vi "BallShear_DependencyCheck.vi"(10 "Power":bool) -> (2 "Ready":bool)   [LabVIEW 2013]
uses:
  <vilib>/LabVIEW Interface for Arduino/LabVIEW Interface for Arduino.lvlib
panel:
  out "standard error":string
  out "standard output":string
  in  "Path to Script":path
  out "Command":string
  out "source":string
  out "code":i32
  out "status":bool
  in  "Errors":bool[](array[boolean])
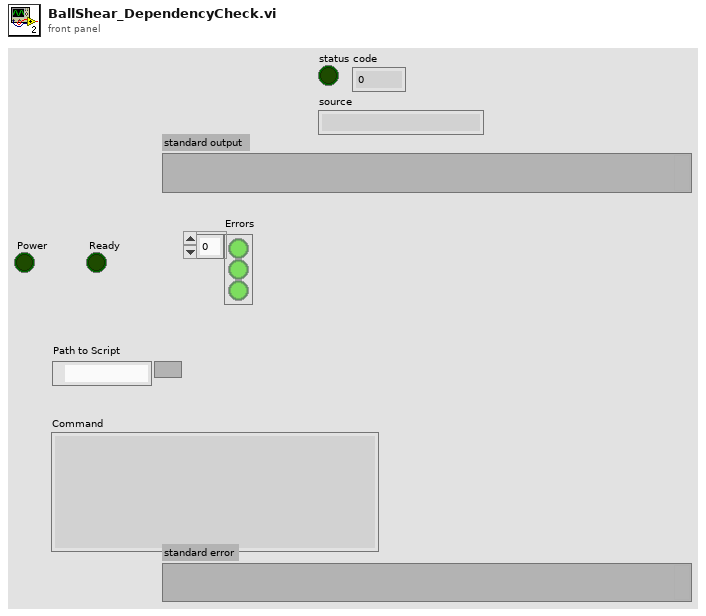
[diagram p1: front panel]
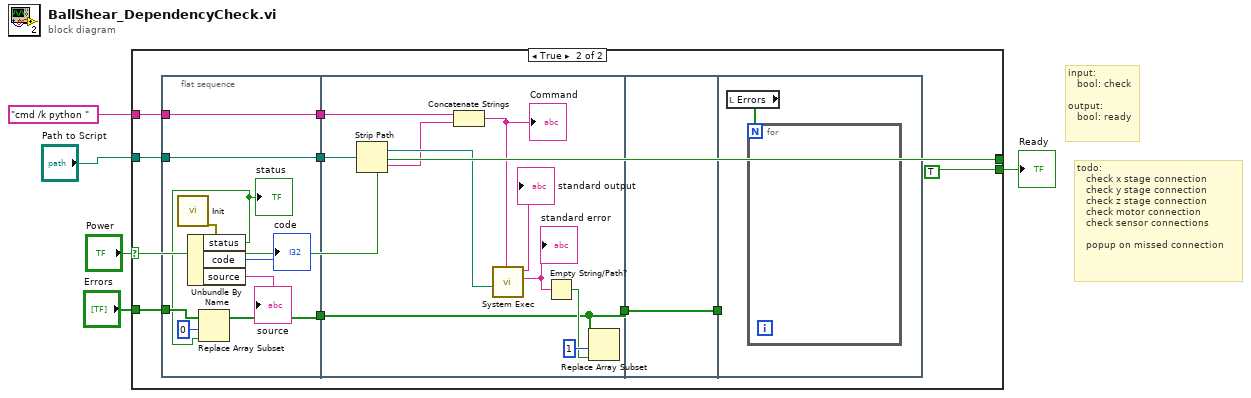
[diagram p0: block diagram]
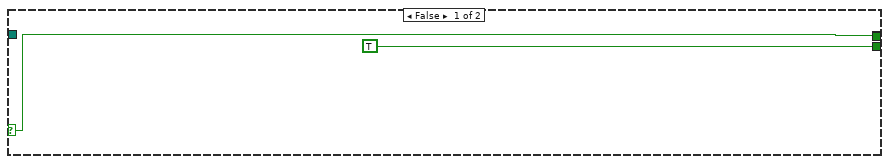
[diagram p2: hidden frame]
diagram:
  # "input:\n   bool: check\n\noutput:\n   bool: ready"
  # "todo:\n   check x stage connection\n   check y stage connection\n   check z stage connection\n   check motor connection\n   check sensor connections\n\n   popup on missed connection"
  n1 = case shown="True" "Power" {
    selector: "Power" -> [w6 _]
    tunnel: [w6 w17] -> _
    tunnel: "Power" -> [_ w17]
    tunnel: [TRUE ("Power") TRUE ("Power")] -> w4
    tunnel: "Errors" -> [_ w14]
    tunnel: "cmd /k python " -> [_ w10]
    tunnel: "Path to Script" -> [_ w9]
    frame False {
    }
    frame True {
      n2 = flat-sequence {
        tunnel: [w22] -> w15
        tunnel: w14 -> [w22]
        tunnel: [w19] -> w11
        tunnel: w10 -> [w19]
        tunnel: w9 -> [w18]
        tunnel: [w18] -> w8
        tunnel: w15 -> [w26]
        tunnel: [w26] -> w12
        tunnel: w11 -> [w32]
        tunnel: w8 -> [w31]
        tunnel: [w36] -> w13
        tunnel: w12 -> [w36]
        tunnel: w13 -> [_]
        frame #0 {
          n3 = call <vilib>:"Init.vi"() -> ("error out"=w25:errorcluster)  [unwired: 18 in, 1 out]
          n4 = Unbundle By Name(w25) -> ("status"=w20:bool, "code"=→"code":i32, "source"=→"source":string)
          "status" <- w20
          n5 = Replace Array Subset(array=w22, new element=w20, index=0) -> ()  [unwired: 1 out]
        }
        frame #1 {
          n6 = Strip Path(path=w31) -> (stripped path=w35:path, name=w33:string)
          n7 = Concatenate Strings(w32, w33) -> (w34:string)
          "Command" <- w34
          n8 = call <vilib>:"System Exec.vi"("working directory"=w35, "command line"=w34) -> ("standard error"=w29:string, "standard output"=→"standard output":string)  [unwired: 6 in, 2 out]
          "standard error" <- w29
          n9 = Empty String/Path?(string/path=w29) -> (empty?=w27:bool)
          n10 = Replace Array Subset(array=w26, new element=w27, index=1) -> ()  [unwired: 1 out]
        }
        frame #2 {
        }
        frame #3 {
          n11 = local read "Errors"() -> (w37:bool[])
          n12 = for {
            N: w37 -> [_]
          }
        }
      }
    }
  }
  "Ready" <- w4
